vi "Find Region Peak Valley Location.vi"(3 "Region Points":cluster{"Y":i32, "X":i32}[](array[cluster]), 4 "Depth Values":dbl[][](array[numeric])) -> (0 "Valley Point Location":cluster{"Y":i32, "X":i32}, 1 "Peak Point Location":cluster{"Y":i32, "X":i32})   [LabVIEW 2018, in "Video Cam Processor.lvclass"]
uses:
  Video Cam Processor.lvclass
  c39c46e9-77d8-4cbc-a29f-2c22cc5b7b36.vi
  c39c46e9-77d8-4cbc-a29f-2c22cc5b7b36.vi/7b002a71-c4fc-441a-adf9-a28fc8f529ae.vi
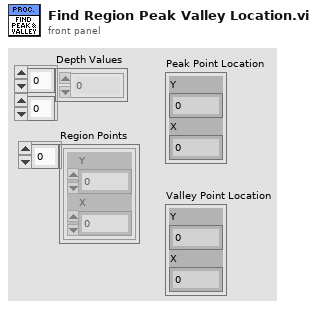
[diagram p1: front panel]
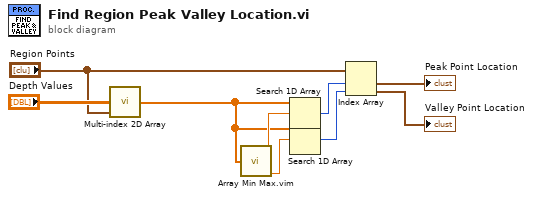
[diagram p0: block diagram]
diagram:
  n1 = call "Multi-index 2D Array.vi"("Indices"="Region Points", "Array"="Depth Values") -> ("Values"=w2:dbl[])  [unwired: 1 in]
  n2 = call "Array Min Max.vim"("Array"=w2) -> ("Max"=w9:dbl, "Min"=w8:dbl)  [unwired: 13 in]
  n3 = Search 1D Array(1D array=w2, element=w9) -> (index of element=w7:i32)  [unwired: 1 in]
  n4 = Search 1D Array(1D array=w2, element=w8) -> (index of element=w6:i32)  [unwired: 1 in]
  n5 = Index Array(array="Region Points", index #1=w7, index #2=w6) -> (element #1=→"Peak Point Location":cluster{"Y":i32, "X":i32}, element #2=→"Valley Point Location":cluster{"Y":i32, "X":i32})
